vi "Initialize.vi"(6 "ID Query (True)":bool=TRUE, 7 "Reset(True)":bool=TRUE, 8 "error in (no error)":errorcluster, 10 "Configuration":T1={"Address"=6, "Baud Rate"=9600, "Language Selector"=1} {"Language Selector" items=["GEN", "SCPI"]; "Baud Rate" items=["1200"=1200, "2400"=2400, "4800"=4800, "9600"=9600, "19200"=19200, "38400"=38400, "57600"=57600, "115200"=115200]}, 11 "VISA resource name":refnum<visa-resource-name>) -> (0 "error out":errorcluster, 3 "VISA resource name out":refnum<visa-resource-name>)   [LabVIEW 2018, in "TDK-Lambda Z.lvlib"]
doc: "Establishes communication with the instrument and optionally performs an instrument identification query and/or an instrument reset. It also places the instrument in a default state needed for other instrument driver operations. Therefore, call this VI before calling other instrument driver VIs for this instrument. Generally, you need to call the <b>Initialize</b> VI only once at the beginning of an application.\n\nThis VI passes the addressing information in the instrument decriptor to the Instr Open VI and returns the instrument ID. You must run this VI before using any of the instrument driver VIs for this instrument."
uses:
  TDK-Lambda Z.lvlib
panel:
  # "(c) 2014-2015 TDK-Lambda.  ALL RIGHTS RESERVED."
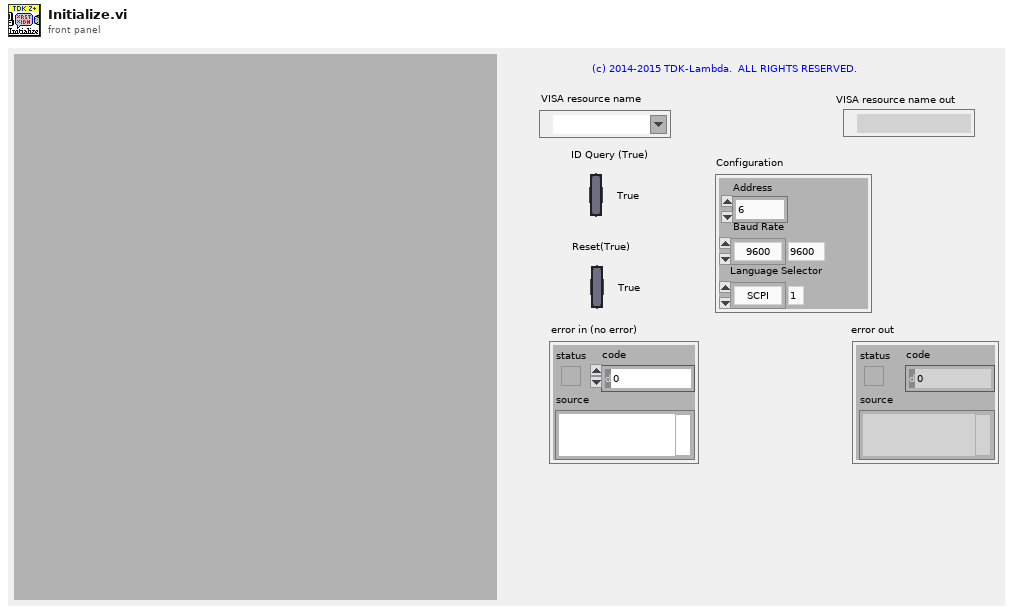
[diagram p1: front panel]
types:
  T1 = cluster{"Address":i16, "Baud Rate":u32, "Language Selector":i16}
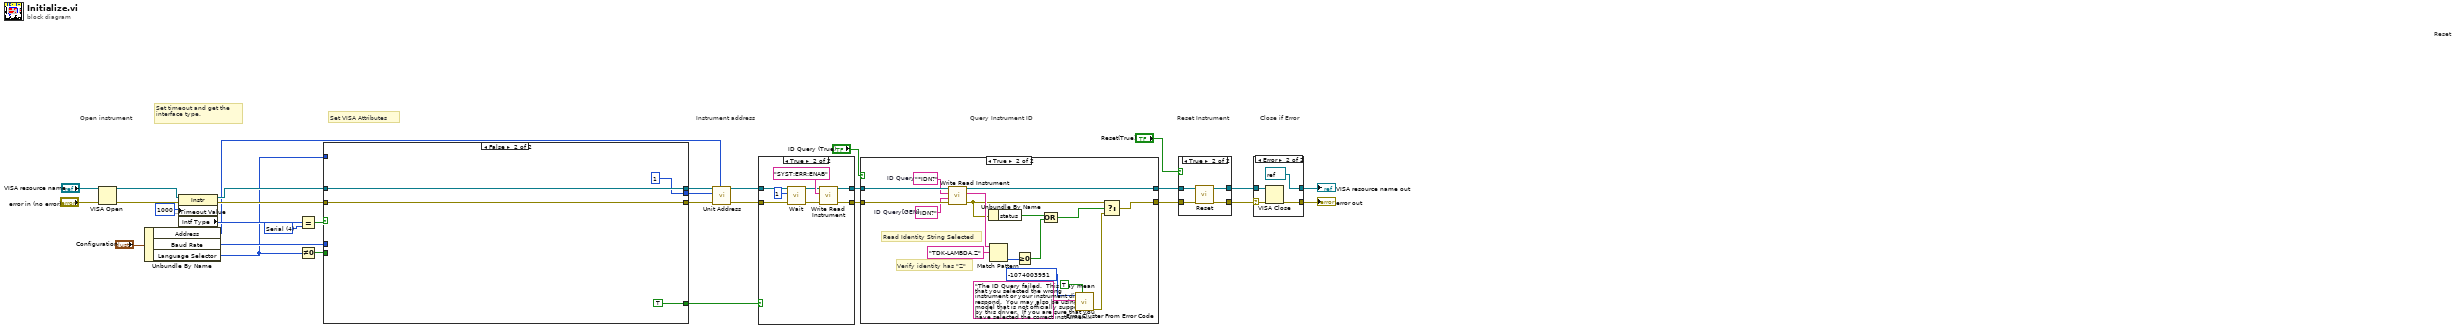
[diagram p0: block diagram]
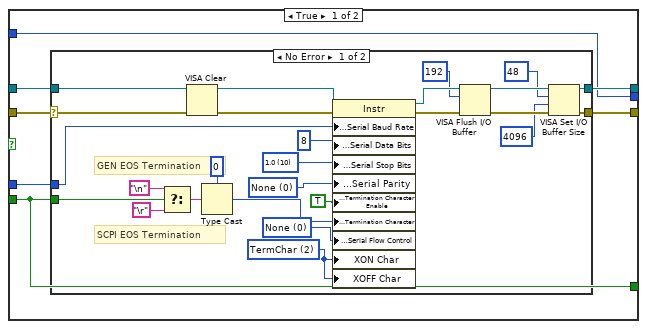
[diagram p6: hidden frame]
diagram:
  w29 = u16 4 items=["GPIB"=1, "VXI"=2, "GPIB-VXI"=3, "Serial"=4, "PXI"=5, "TCPIP"=6, "USB"=7] ("Interface Information:Interface Type")
  # "Query Instrument ID"
  # "Reset Instrument"
  # "Close if Error"
  # "Reset"
  # "Set VISA Attributes"
  # "Instrument address"
  # "Set timeout and get the\ninterface type."
  # "Open instrument"
  n1 = VISA Open(error in (no error)="error in (no error)", VISA resource name="VISA resource name") -> (VISA resource name=w2:refnum<visa-resource-name>, error out=w1:errorcluster)  [unwired: 3 in]
  n2 = Unbundle By Name("Configuration") -> ("Address"=w3:i16, "Baud Rate"=w6:u32, "Language Selector"=w5:i16)
  n3 = property class="Instr"(reference=w2, error in=w1, "General Settings:Timeout Value"=u32 1000 ("Tmo Value")) -> (reference out=w30:refnum<visa-resource-name>, error out=w31:errorcluster, "Intf Type"=w28:u16)
  n4 = Equal?(x=w28, y=w29) -> (x = y?=w27:bool)
  n5 = Not Equal To 0?(x=w5) -> (x != 0?=w18:bool)
  n6 = case shown="False" w27 {
    tunnel: w31 -> [w35 w69]
    tunnel: w30 -> [w38 w70]
    tunnel: [w37 w70] -> w26
    tunnel: [w36 w69] -> w25
    tunnel: [w33 TRUE] -> w17
    tunnel: w18 -> [w33 _]
    tunnel: w5 -> [w34 _]
    tunnel: [w34 i16 1 ("Language Selector")] -> w4
    tunnel: w6 -> [w32 _]
    frame True {
      n7 = case shown="No Error" w35 {
        selector: w35 -> [w41 w66]
        tunnel: w38 -> [w42 w65]
        tunnel: [w56 w65] -> w37
        tunnel: [w55 w66] -> w36
        tunnel: w33 -> [w51 _]
        tunnel: w32 -> [w45 _]
        frame No Error {
          w44 = u16 0 items=["None", "Odd", "Even", "Mark", "Space"] ("Serial Settings:Parity")
          w43 = u8 2 items=["None", "LastBit", "TermChar"] ("Serial Settings:Serial End Mode for Reads")
          w63 = u16 10 items=["1.0"=10, "1.5"=15, "2.0"=20] ("stop bits (10: 1 bit)")
          w61 = u16 0 items=["None", "XON/XOFF", "RTS/CTS", "XON/XOFF & RTS/CTS", "DTR/DSR", "XON/XOFF & DTR/DSR"] ("flow control (0:none)")
          # "SCPI EOS Termination"
          # "GEN EOS Termination"
          n8 = Select(t="\n", s=w51, f="\r") -> (s? t:f=w54:string)
          n9 = VISA Clear(VISA resource name=w42, error in (no error)=w41) -> (VISA resource name out=w40:refnum<visa-resource-name>, error out=w39:errorcluster)
          n10 = Type Cast(type=u8 0, x=w54) -> (*(type *) &x=w59:u8)
          n11 = property class="Instr"(reference=w40, error in=w39, "Serial Settings:Serial Baud Rate"=w45, "Serial Settings:Serial Data Bits"=u16 8 ("data bits (8)"), "Serial Settings:Serial Stop Bits"=w63, "Serial Settings:Serial Parity"=w44, "Message Based Settings:Termination Character Enable"=TRUE ("Enable Termination\nChar (T)"), "Message Based Settings:Termination Character"=w59, "Serial Settings:Serial Flow Control"=w61, "XON Char"=w43, "XOFF Char"=w43) -> (reference out=w57:refnum<visa-resource-name>, error out=w58:errorcluster)
          n12 = VISA Flush I/O Buffer(VISA resource name=w57, mask (16)=u16 192, error in (no error)=w58) -> (VISA resource name out=w50:refnum<visa-resource-name>, error out=w49:errorcluster)
          n13 = VISA Set I/O Buffer Size(VISA resource name=w50, mask (16)=u16 48, size (4096)=u32 4096 ("size (0)"), error in (no error)=w49) -> (VISA resource name out=w56:refnum<visa-resource-name>, error out=w55:errorcluster)
        }
        frame Error {
        }
      }
    }
    frame False {
    }
  }
  n14 = call "Unit Address.vi"("Address (6)"=w3, "error in (no error)"=w25, "Language Selector (-1)"=w4, "VISA resource name"=w26) -> ("error out"=w22:errorcluster, "VISA resource name out"=w23:refnum<visa-resource-name>)  [unwired: 6 in]
  n15 = case shown="True" w17 {
    tunnel: w23 -> [w72 w77]
    tunnel: w22 -> [w71 w78]
    tunnel: [w72 w74] -> w21
    tunnel: [w71 w73] -> w20
    frame False {
    }
    frame True {
      n16 = call "Wait.vi"("error in (no error)"=w78, "Wait (1mS)"=u32 1 ("Delay (1 mS)"), "VISA resource name"=w77) -> ("error out"=w75:errorcluster, "VISA resource name out"=w76:refnum<visa-resource-name>)  [unwired: 7 in]
      n17 = call "Write Read Instrument.vi"("error in (no error)"=w75, "SCPI  Write Command/Query"="SYST:ERR:ENAB" ("Write Command/Query"), "VISA resource name"=w76) -> ("error out"=w73:errorcluster, "VISA resource name out"=w74:refnum<visa-resource-name>)  [unwired: 6 in, 1 out]
    }
  }
  n18 = case shown="True" "ID Query (True)" {
    tunnel: w21 -> [w82 w99]
    tunnel: w20 -> [w81 w98]
    tunnel: [w82 w97] -> w14
    tunnel: [w81 w91] -> w15
    frame False {
    }
    frame True {
      w89 = "*IDN?"  # ID Query
      w88 = "IDN?"  # ID Query[GEN]
      # "Verify identity has \"Z\""
      # "Read Identity String Selected"
      n19 = call "Write Read Instrument.vi"("error in (no error)"=w98, "GEN  Write Command/Query"=w88, "SCPI  Write Command/Query"=w89, "VISA resource name"=w99) -> ("error out"=w87:errorcluster, "Response"=w90:string, "VISA resource name out"=w97:refnum<visa-resource-name>)  [unwired: 5 in]
      n20 = Unbundle By Name(w87) -> ("status"=w84:bool)
      n21 = Match Pattern(string=w90, regular expression="TDK-LAMBDA,Z") -> (offset past match=w86:i32)  [unwired: 1 in, 3 out]
      n22 = Greater Or Equal To 0?(x=w86) -> (x >= 0?=w85:bool)
      n23 = Compound Arithmetic op=OR(w84, w85) -> (w83:bool)
      n24 = call <vilib>:"Error Cluster From Error Code.vi"("show call chain? (False)"=TRUE, "error message (\"\")"="The ID Query failed.  This may mean that you selected the wrong instrument or your instrument did not respond.  You may also be using a model that is not officially supported by this driver.  If you are sure that you have selected the correct instrument and it is responding, try disabling the ID Query." ("Source (VI Name)"), "error code (0)"=-1074003951 ("Code")) -> ("error out"=w92:errorcluster)  [unwired: 6 in]
      n25 = Select(t=w87, s=w83, f=w92) -> (s? t:f=w91:errorcluster)
    }
  }
  n26 = case shown="True" "Reset(True)" {
    tunnel: w15 -> [w100 w105]
    tunnel: w14 -> [w101 w104]
    tunnel: [w101 w103] -> w13
    tunnel: [w100 w102] -> w12
    frame False {
    }
    frame True {
      n27 = call "Reset.vi"("error in (no error)"=w105, "VISA resource name"=w104) -> ("error out"=w102:errorcluster, "VISA resource name out"=w103:refnum<visa-resource-name>)  [unwired: 8 in]
    }
  }
  n28 = case shown="Error" w12 {
    selector: w12 -> [w107 w111]
    tunnel: w13 -> [w106 w109]
    tunnel: [w107 w110] -> w7
    tunnel: [w106 refnum<visa-resource-name> refnum ("VISA resource name out")] -> w10
    frame No Error {
    }
    frame Error {
      n29 = VISA Close(VISA resource name=w109, error in (no error)=w111) -> (error out=w110:errorcluster)
    }
  }
  "VISA resource name out" <- w10
  "error out" <- w7
